vi "Core Action.vi"(8 "error in (no error)":errorcluster, 10 "SECS-II Class":refnum<class "SECS-II Class.lvclass">, 11 "05-Host Send Equipment Constant Values in":refnum<class "05-Host Send Equipment Constant Values.lvclass">) -> (0 "error out":errorcluster, 2 "SECS-II Class Out":refnum<class "SECS-II Class.lvclass">, 3 "05-Host Send Equipment Constant Values out":refnum<class "05-Host Send Equipment Constant Values.lvclass">)   [LabVIEW 2020, in "SECS Scenarios.lvlib" / "05-Host Send Equipment Constant Values.lvclass"]
uses:
  05-Host Send Equipment Constant Values.lvclass
  D:/Dropbox/SECS/SECS_GEM v1.1.0/Com/SECS Scenarios/Scenarios Class/Scenarios Class.lvclass
  SECS Communication/SECS-II Class/SECS-II Class.lvclass
  SECS Communication/S2 Message Class/S2 Message Class.lvclass
  D:/Dropbox/SECS/SECS_GEM v1.1.0/Com/SECS Communication/SECS-II Class/SECS-II Class.lvclass
  Scenarios Class/Reply State.ctl
  Scenarios Class/Scenarios Class.lvclass/Scenarios Class.ctl
  SECS Communication/S2 Message Class/S2F16.ctl
  Scenarios Class/Write Reply State.vi
  Scenarios Class/Read HSMS Class.vi
  SECS Communication/SECS Data Class/Get ECID Data.vi
  SECS Communication/SECS Data Class/Put ECID Data.vi
  SECS Communication/HSMS Class/HSMS Class.lvclass
  SECS Communication/SECS Data Class/SECS Data Class.lvclass
  Scenarios Class/Scenarios Class.lvclass
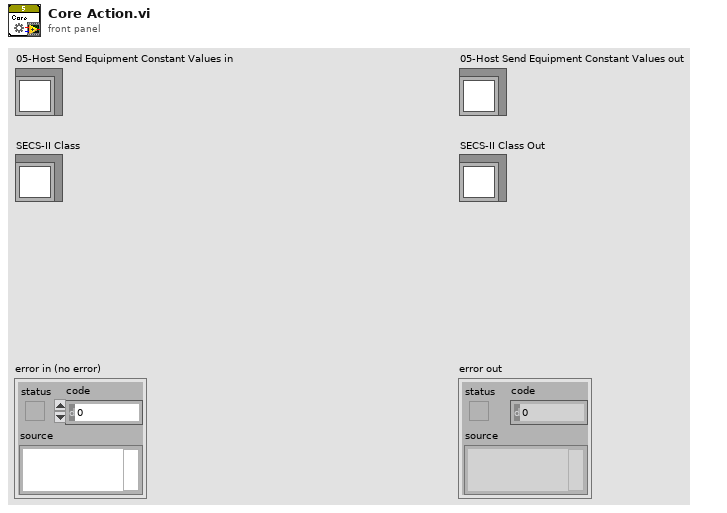
[diagram p1: front panel]
types:
  T1 = typedef "SECS Communication.lvlib/S2 Message Class.lvclass/S2F15.ctl" = cluster{"ECID":u32, "ECV":cluster{"Format Code":T2, "Value":variant}}[]
  T2 = typedef "SECS Communication.lvlib/SECS-II Class.lvclass/Format Code.ctl" = enum16{"L", "A", "B", "Boolean", "J", "I1", "I2", "I4", "I8", "U1", "U2", "U4", "U8", "F4", "F8", "Char"}
  T3 = typedef "SECS Scenarios.lvlib/Scenarios Class.lvclass/Reply State.ctl" = enum16{"OK", "Illegal Data", "Unknown Stream", "Unknown Function", "Off-Line", "T3 Timeout", "Inner-Timeout"}
  T4 = typedef "SECS Communication.lvlib/S2 Message Class.lvclass/S2F16.ctl" = enum16{"OK", "one or more constants does not exist", "busy", "one or more values out of range"}
  T5 = typedef "SECS Communication.lvlib/SECS Data Class.lvclass/ECID Data.ctl" = cluster{"ECID":u32, "Name":string, "Description":string, "Format Code":T2, "Unit":string, "Max":dbl, "Min":dbl, "Default":string, "Source":string, "Data":variant}
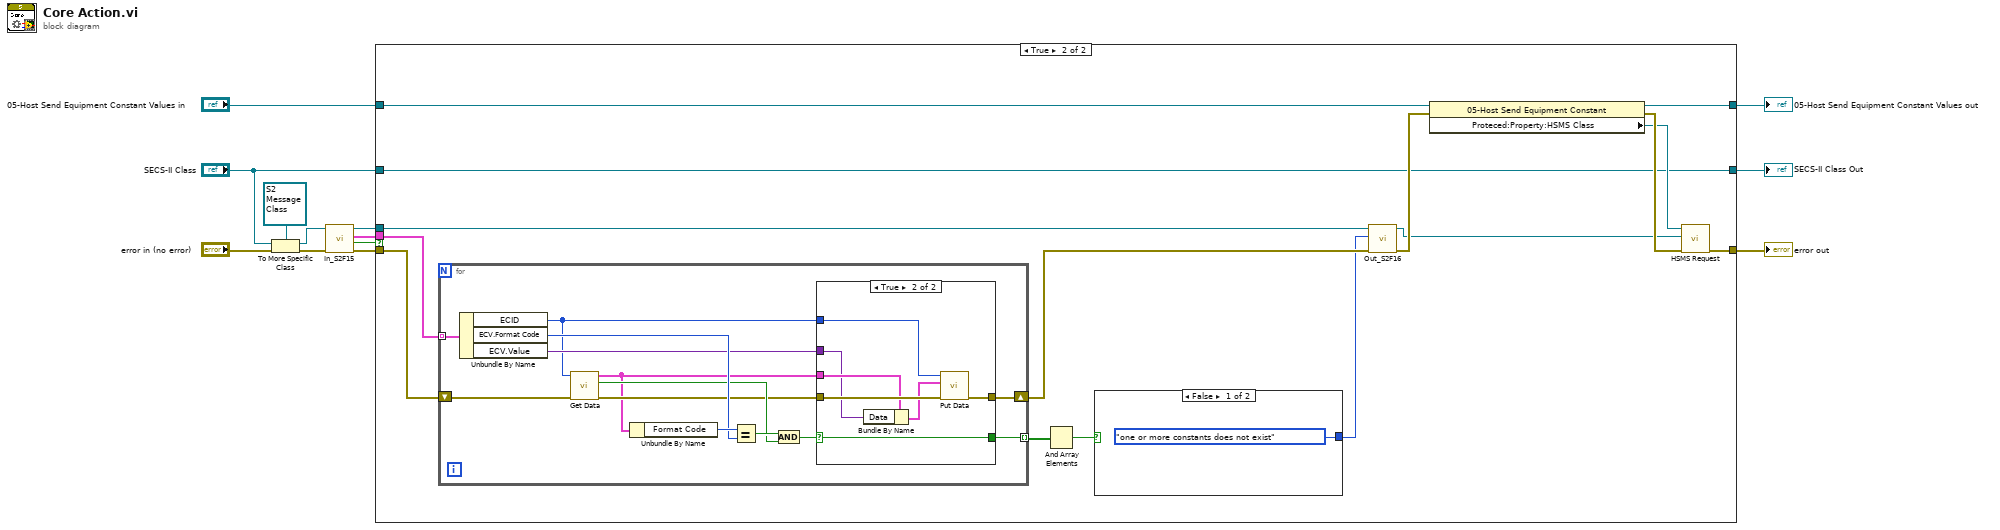
[diagram p0: block diagram]
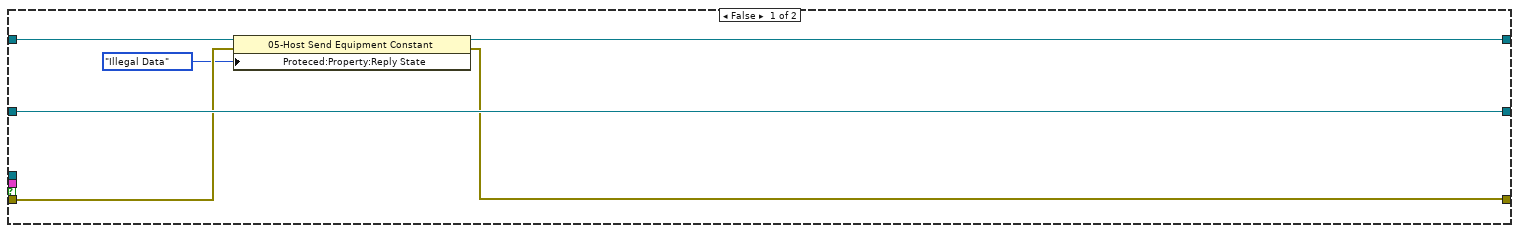
[diagram p2: hidden frame]
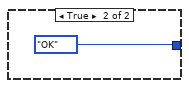
[diagram p3: hidden frame]
diagram:
  n1 = To More Specific Class(target class=refnum<class "S2 Message Class.lvclass"> refnum ("SECS Communication.lvlib:S2 Message Class.lvclass"), reference="SECS-II Class", error in="error in (no error)") -> (specific class reference=w10:refnum<class "S2 Message Class.lvclass">, error out=w11:errorcluster)
  n2 = call "In_S2F15.vi"("error in (no error)"=w11, "S2 Message Class in"=w10) -> ("error out"=w9:errorcluster, "OK?"=w3:bool, "S2F15"=w8:T1, "S2 Message Class out"=w7:refnum<class "S2 Message Class.lvclass">)  [unwired: 6 in]
  n3 = case shown="True" w3 {
    tunnel: w9 -> [w17 w34]
    tunnel: w8 -> [_ w33]
    tunnel: w7 -> [_ w31]
    tunnel: "05-Host Send Equipment Constant Values in" -> [w18 w27]
    tunnel: [w15 w22] -> w5
    tunnel: [w14 w21] -> w4
    tunnel: "SECS-II Class" -> [w19 w20]
    tunnel: [w19 w20] -> w1
    frame False {
      n4 = property class="05-Host Send Equipment Constant"(reference=w18, error in=w17, "Proteced:Property:Reply State"=Reply_State."Illegal Data" ("Reply State")) -> (reference out=w15:refnum<class "05-Host Send Equipment Constant Values.lvclass">, error out=w14:errorcluster)
    }
    frame True {
      n5 = for {
        shift-right: [w38] -> w29
        shift-left: w34 -> [w49]
        tunnel: w33 -> [w48] mode=indexing
        tunnel: [w37] -> w32 mode=indexing
        n6 = Unbundle By Name(w48) -> ("ECID"=w39:u32, "ECV.Format Code"=w46:T2, "ECV.Value"=w41:variant)
        n7 = call-poly "Get Data.vi"("error in"=w49, "ECID"=w39) -> ("error out"=w42:errorcluster, "Find?"=w44:bool, "ECID Data"=w40:T5)  [unwired: 7 in]
        n8 = Unbundle By Name(w40) -> ("Format Code"=w47:T2)
        n9 = Equal?(x=w47, y=w46) -> (x = y?=w45:bool)
        n10 = And(x=w45, y=w44) -> (x .and. y?=w43:bool)
        n11 = case shown="True" w43 {
          selector: w43 -> [w50 w52]
          tunnel: w42 -> [w51 w58]
          tunnel: w41 -> [_ w56]
          tunnel: w40 -> [_ w57]
          tunnel: w39 -> [_ w54]
          tunnel: [w51 w53] -> w38
          tunnel: [w50 w52] -> w37
          frame False {
          }
          frame True {
            n12 = Bundle By Name(cluster=w57, "Data"=w56) -> (w55:T5)
            n13 = call-poly "Put Data.vi"("error in"=w58, "ECID Data"=w55, "ECID"=w54) -> ("error out"=w53:errorcluster)  [unwired: 7 in, 1 out]
          }
        }
      }
      n14 = And Array Elements(Boolean array=w32) -> (logical AND=w30:bool)
      n15 = case shown="False" w30 {
        tunnel: [S2F16."one or more constants does not exist" ("S2F16") S2F16."OK" ("S2F16")] -> w28
        frame False {
        }
        frame True {
        }
      }
      n16 = call "Out_S2F16.vi"("error in (no error)"=w29, "S2F16"=w28, "S2 Message Class in"=w31) -> ("error out"=w26:errorcluster, "S2 Message Class out"=w24:refnum<class "S2 Message Class.lvclass">)  [unwired: 7 in]
      n17 = property class="05-Host Send Equipment Constant"(reference=w27, error in=w26) -> (reference out=w22:refnum<class "05-Host Send Equipment Constant Values.lvclass">, error out=w25:errorcluster, "Proteced:Property:HSMS Class"=w23:refnum<class "HSMS Class.lvclass">)
      n18 = call "HSMS Request.vi"("error in (no error)"=w25, "SECS-II Class In"=w24, "HSMS Class in"=w23) -> ("error out"=w21:errorcluster)  [unwired: 7 in, 1 out]
    }
  }
  "error out" <- w4
  "05-Host Send Equipment Constant Values out" <- w5
  "SECS-II Class Out" <- w1
